vi "Test Alt Async.vi"() -> ()   [LabVIEW 2013]
uses:
  alt Ctl Ref.ctl
panel:
  in  "Stop":bool
  out "AltSP":i32
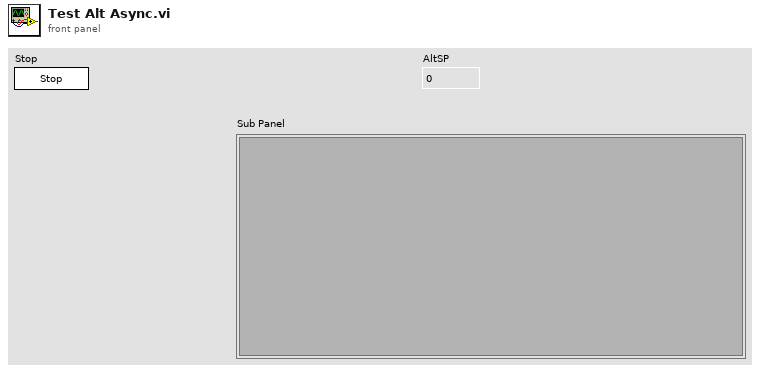
[diagram p1: front panel]
types:
  T1 = typedef "alt Ctl Ref.ctl" = refnum<vi>
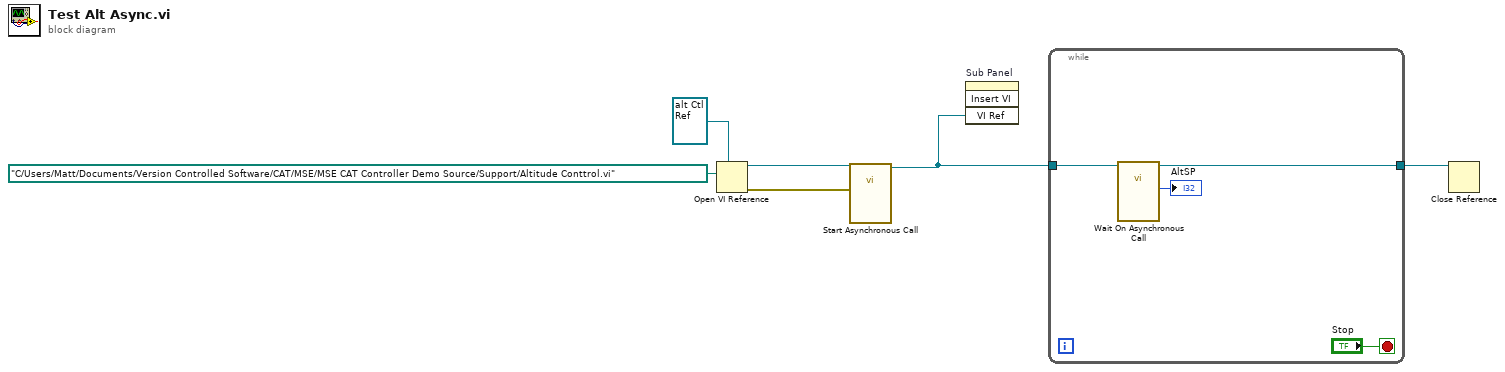
[diagram p0: block diagram]
diagram:
  n1 = Open VI Reference(type specifier VI Refnum (for type only)=T1 refnum, vi path=path "C:/Users/Matt/Documents/Version Controlled Software/CAT/MSE/MSE CAT Controller Demo Source/Support/Altitude Conttrol.vi") -> (vi reference=w5:T1, error out=w4:errorcluster)  [unwired: 4 in]
  n2 = call-by-ref "Start Asynchronous Call"(reference=w5, error in=w4) -> (reference out=w3:T1)  [unwired: 11 in, 2 out]
  n3 = invoke on="Sub Panel" class="SubPanel" method="Insert VI"("VI Ref"=w3) -> ()  [unwired: 3 in, 4 out]
  n4 = while {
    tunnel: w3 -> [w10]
    tunnel: [w7] -> w1
    stop <- "Stop" stop-if-true
    n5 = call-by-ref "Wait On Asynchronous Call"(reference=w10) -> (reference out=w7:T1, "AltSP"=→"AltSP":i32)  [unwired: 12 in, 1 out]
  }
  n6 = Close Reference(reference=w1) -> ()  [unwired: 1 in, 1 out]
